vi "GenerateDC.vi"(1 "DC value":dbl caption="Offset") -> (0 "Signal":dynamicdata(graph) caption="DC")   [LabVIEW 2014]
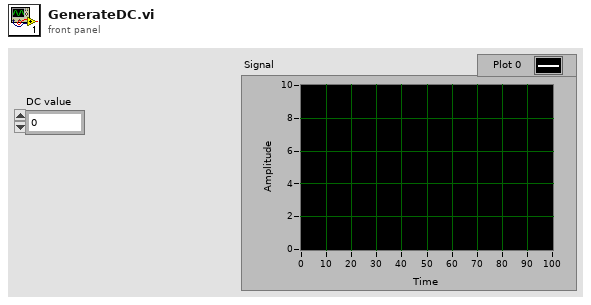
[diagram p1: front panel]
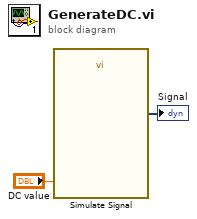
[diagram p0: block diagram]
diagram:
  n1 = call "Simulate Signal"("Offset"="DC value") -> ("DC"=→"Signal":dynamicdata)  [unwired: 13 in, 1 out]
